vi "Sims Vision Method.vi"(1 "Vert Theta (0.375)":dbl, 2 "Image Hight In Pixels":dbl, 3 "Offset":dbl, 4 "Target Height In Inches":dbl, 5 "Target Hight In Pixels":dbl, 6 "FOV Angle":dbl) -> (0 "Distance":dbl)   [LabVIEW 2015]
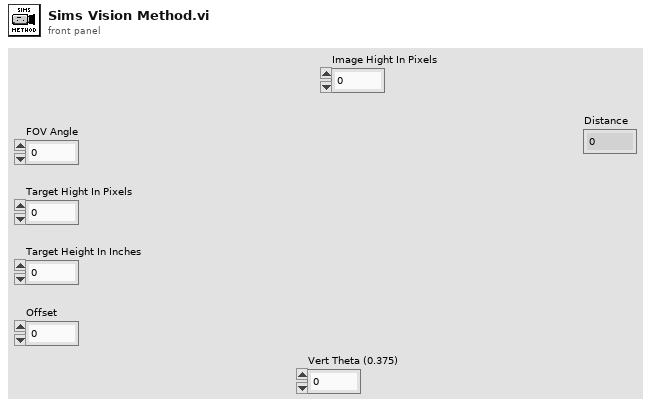
[diagram p1: front panel]
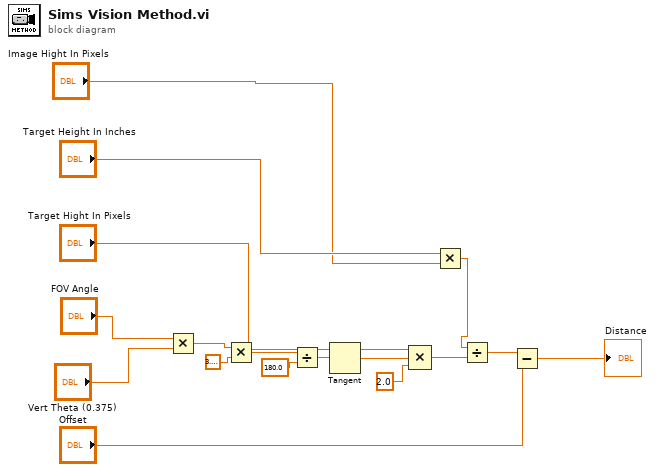
[diagram p0: block diagram]
diagram:
  n1 = Multiply(x="FOV Angle", y="Vert Theta (0.375)") -> (x*y=w16:dbl)
  n2 = Multiply(x=w16, y=3.141592653589793) -> (x*y=w14:dbl)
  n3 = Divide(x=w14, y=180.0) -> (x/y=w12:dbl)
  n4 = Tangent(1:w12) -> (0:w11:dbl)
  n5 = Compound Arithmetic op=MULTIPLY("Target Hight In Pixels", w11, 2.0 ("value")) -> (w8:dbl)
  n6 = Multiply(x="Target Height In Inches", y="Image Hight In Pixels") -> (x*y=w5:dbl)
  n7 = Divide(x=w5, y=w8) -> (x/y=w4:dbl)
  n8 = Subtract(x=w4, y="Offset") -> (x-y=→"Distance":dbl)
